vi "about.vi"(8 "更新包远端地址":string="/UP/OneStation/V4/一体化微型水质监测站.zip", 9 "SN输入":string="SN", 10 "站点名称输入":string="站点名称", 11 "应用程序名称输入":string="地表水水质自动监测系统") -> ()   [LabVIEW 2016, in "数据传输系统-04.lvlib" / "update.lvlib"]
uses:
  update.lvlib
  <vilib>/Utility/miscctls.llb/LVPointTypeDef.ctl
panel:
  in  "正式版/测试版":bool
  in  "检查更新":bool
  in  "更新日志":bool
  out "SN":string="SN"
  out "站点名称":string="站点名称"
  out "Version":string="Version 1.0.0"
  out "应用程序名称":string="地表水水质自动监测系统"
  # "关于"
  # "软件名称:"
  # "软件版本:"
  # "站点名称:"
  # "序列号:"
  # "Copyright (c) 2019. All rights reserved."
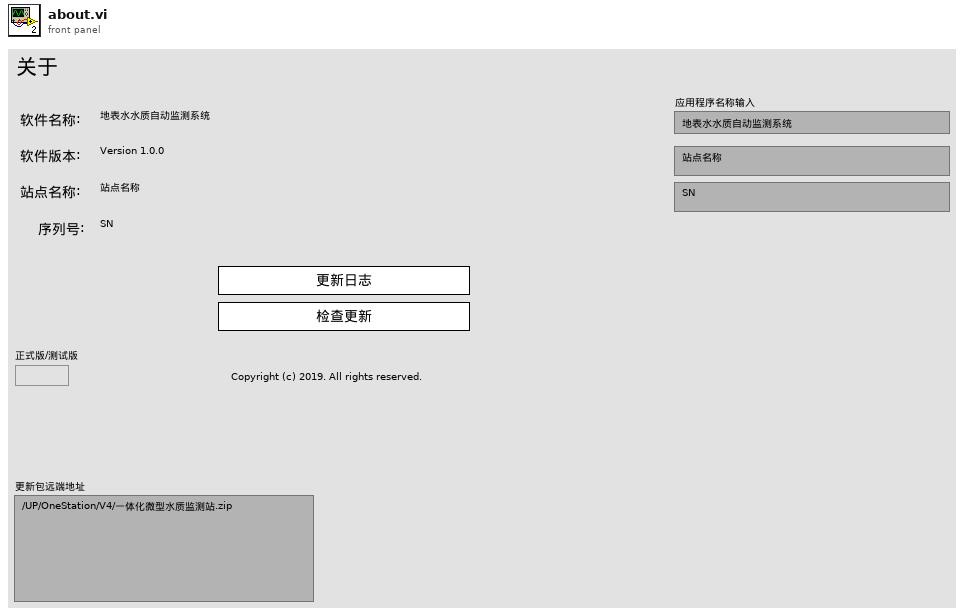
[diagram p1: front panel]
types:
  T1 = typedef "LVPointTypeDef.ctl" = cluster{"Horizontal":i16, "Vertical":i16}
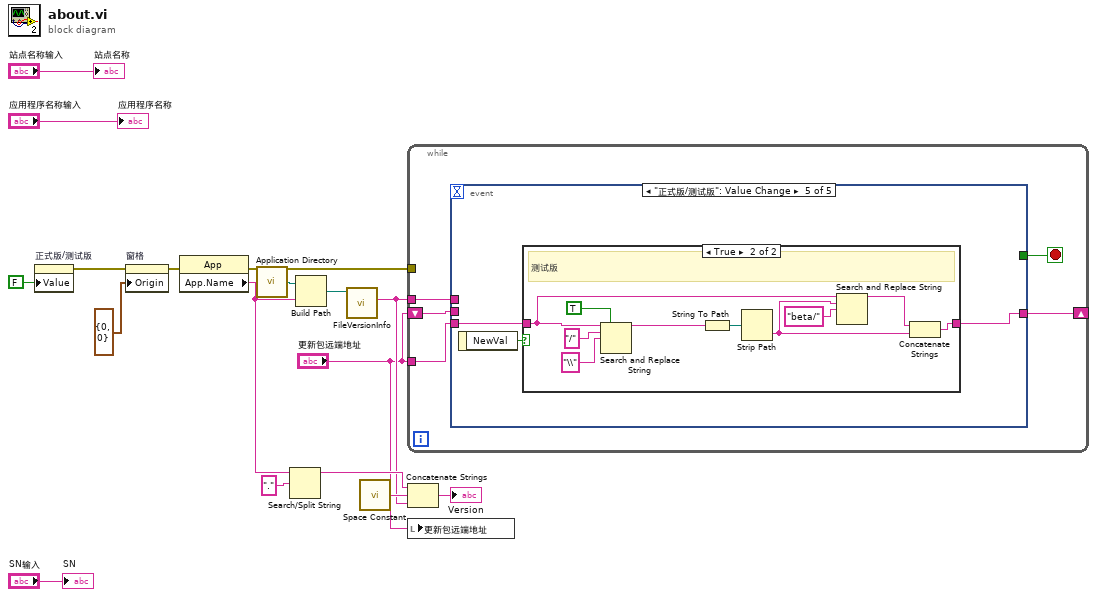
[diagram p0: block diagram]
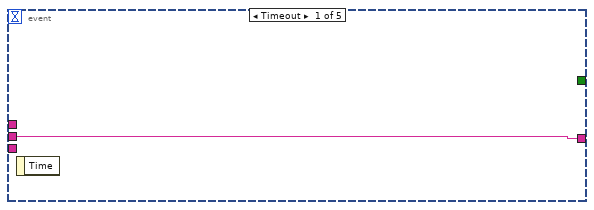
[diagram p2: hidden frame]
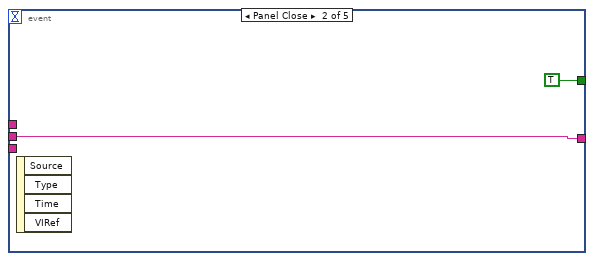
[diagram p3: hidden frame]
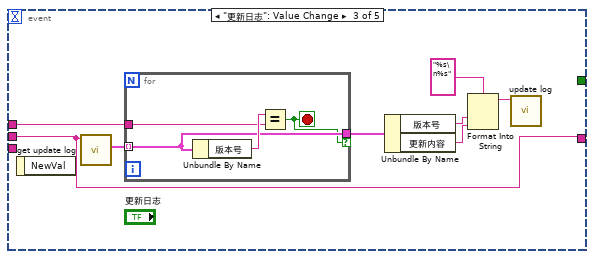
[diagram p4: hidden frame]
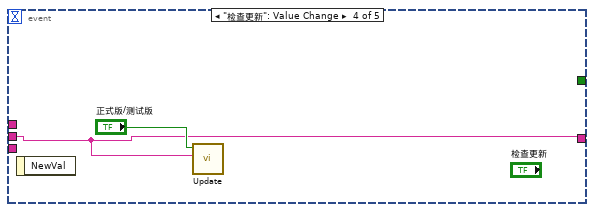
[diagram p5: hidden frame]
diagram:
  n1 = property on="正式版/测试版" class="Bool (strict)"("Value"=FALSE ("正式版/测试版")) -> (error out=w4:errorcluster)  [unwired: 2 in, 1 out]
  n2 = property on="窗格" class="Pane"(error in=w4, "Origin"=T1 {"Horizontal"=0, "Vertical"=0} ("原点")) -> (error out=w7:errorcluster)  [unwired: 1 in, 1 out]
  n3 = property class="App"(error in=w7) -> (error out=w6:errorcluster, "App.Name"=w16:string)  [unwired: 1 in, 1 out]
  n4 = call <vilib>:"Application Directory.vi"() -> ("Application Directory"=w3:path)
  n5 = Search/Split String(string=w16, search string/char (-)="." ("搜索字符串/字符(-)")) -> (substring before match=w8:string)  [unwired: 1 in, 2 out]
  n6 = Build Path(base path=w3, name or relative path=w16) -> (appended path=w14:path)
  n7 = call <vilib>:"FileVersionInfo.vi"("Application Path in"=w14) -> ("File Version Info"=w2:string)  [unwired: 7 in, 3 out]
  n8 = call <vilib>:"Space Constant.vi"() -> ("String"=w12:string)
  n9 = while {
    tunnel: w6 -> [_]
    tunnel: "更新包远端地址" -> [w21]
    shift-right: [w20] -> _
    shift-left: "更新包远端地址" -> [w19]
    tunnel: w2 -> [w18]
    stop <- w22 stop-if-true
    n10 = event shown="[4] \"正式版/测试版\": Value Change" {
      selector: _ -> [_ _ _ _ _]
      dyn-events: _ -> [_ _ _ _ _]
      timeout: _ -> [_ _ _ _ _]
      tunnel: [_ TRUE _ _ _] -> w22
      tunnel: [w23 w24 w27 w38 w41] -> w20
      tunnel: w21 -> [_ _ _ _ w40]
      tunnel: w19 -> [w23 w24 w27 w38 _]
      tunnel: w18 -> [_ _ w29 _ _]
      event Timeout {
        n11 = event-data() -> ()  [unwired: 1 in, 1 out]
      }
      event Panel Close {
        n12 = event-data() -> ()  [unwired: 1 in, 4 out]
      }
      event "更新日志": Value Change {
        n13 = event-data() -> ()  [unwired: 1 in, 1 out]
        n14 = call "get update log.vi"("远端地址"=w27) -> ("版本信息"=w26:cluster{"版本号":string, "更新内容":string}[])  [unwired: 8 in, 2 out]
        n15 = for {
          tunnel: w26 -> [w35] mode=indexing
          tunnel: w29 -> [w36]
          tunnel: [w35] -> w28 if=w34
          stop <- w34 stop-if-true
          n16 = Unbundle By Name(w35) -> ("版本号"=w37:string)
          n17 = Equal?(x=w37, y=w36) -> (x = y?=w34:bool)
        }
        n18 = Unbundle By Name(w28) -> ("版本号"=w32:string, "更新内容"=w31:string)
        n19 = Format Into String(format string="%s\n%s" ("格式字符串"), w32, w31) -> (resulting string=w30:string)  [unwired: 2 in, 1 out]
        n20 = call "update log.vi"("更新记录"=w30) -> ()  [unwired: 10 in, 1 out]
      }
      event "检查更新": Value Change {
        n21 = event-data() -> ()  [unwired: 1 in, 1 out]
        n22 = call "Update.vi"("更新包远端地址"=w38, "测试版？"="正式版/测试版") -> ()  [unwired: 10 in]
      }
      event "正式版/测试版": Value Change {
        n23 = event-data() -> ("NewVal"=w42:bool)  [unwired: 1 in]
        n24 = case shown="True" w42 {
          tunnel: [w43 w44] -> w41
          tunnel: w40 -> [w43 w48]
          frame False {
            # "默认正式版"
          }
          frame True {
            # "测试版"
            n25 = Search and Replace String(replace all?=TRUE ("替换全部？(F)"), input string=w48, search string="/" ("分隔符(Tab)"), replace string="\\" ("替换字符串(\"\")")) -> (result string=w50:string)  [unwired: 4 in, 3 out]
            n26 = String To Path(string=w50) -> (path=w49:path)
            n27 = Strip Path(path=w49) -> (name=w45:string)  [unwired: 1 out]
            n28 = Search and Replace String(input string=w48, search string=w45, replace string="beta/" ("字符串")) -> (result string=w46:string)  [unwired: 5 in, 3 out]
            n29 = Concatenate Strings(w46, w45) -> (w44:string)
          }
        }
      }
    }
  }
  n30 = Concatenate Strings(w8, w12, w2) -> (→"Version":string)
  n31 = local write "更新包远端地址"("更新包远端地址") -> ()
  "应用程序名称" <- "应用程序名称输入"
  "站点名称" <- "站点名称输入"
  "SN" <- "SN输入"
